vi "Format XML Parameters in Tree.vi"(7 "Path  Array IN":string[](array[string]), 8 "error in (no error)":errorcluster, 9 "Current path index":i32, 10 "Newly Added Tag":string, 11 "Tree Refnum":refnum<vi>) -> ()   [LabVIEW 2012]
doc: "SciScan 1.2 160622"
panel:
  out "error out":errorcluster
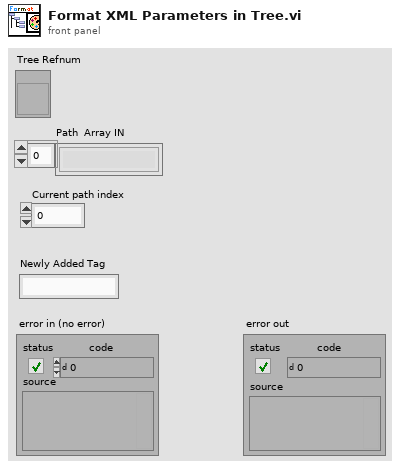
[diagram p1: front panel]
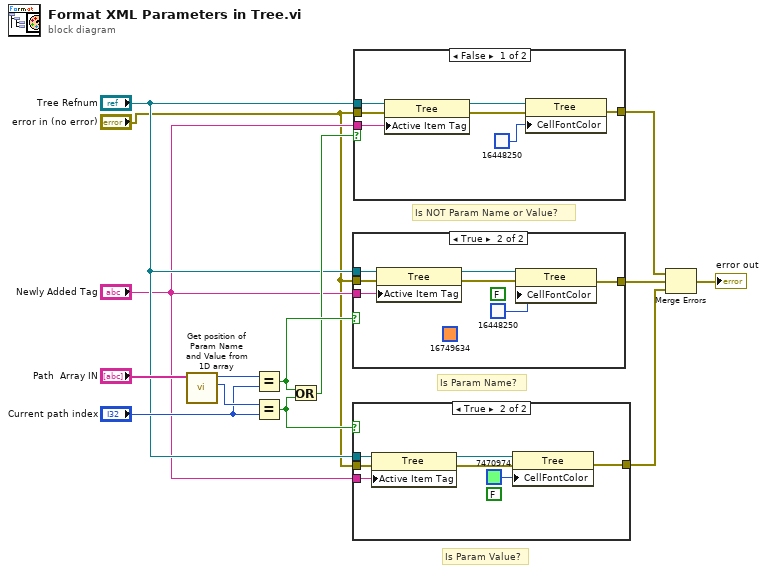
[diagram p0: block diagram]
diagram:
  # "Is NOT Param Name or Value?"
  # "Is Param Name?"
  # "Is Param Value?"
  n1 = call "Get position of Param Name and Value from 1D array.vi"("1D path array"="Path  Array IN") -> ("Index of Param Value"=w12:i32, "Index of Param Name"=w13:i32)  [unwired: 9 in]
  n2 = Equal?(x=w13, y="Current path index") -> (x = y?=w10:bool)
  n3 = Equal?(x=w12, y="Current path index") -> (x = y?=w9:bool)
  n4 = Or(x=w10, y=w9) -> (x .or. y?=w8:bool)
  n5 = case shown="True" w10 {
    tunnel: "Tree Refnum" -> [_ w22]
    tunnel: "Newly Added Tag" -> [_ w21]
    tunnel: "error in (no error)" -> [w15 w20]
    tunnel: [w15 w19] -> w3
    frame False {
    }
    frame True {
      (unwired) u32 16749634
      (unwired) FALSE ("Active Cell:Cell Font:Italic")
      n6 = property class="Tree"(reference=w22, error in=w20, "Active Item Tag"=w21) -> (reference out=w18:refnum<vi>, error out=w17:errorcluster)
      n7 = property class="Tree"(reference=w18, error in=w17, "CellFontColor"=u32 16448250) -> (error out=w19:errorcluster)  [unwired: 1 out]
    }
  }
  n8 = case shown="True" w9 {
    tunnel: "Newly Added Tag" -> [_ w30]
    tunnel: "Tree Refnum" -> [_ w29]
    tunnel: "error in (no error)" -> [w23 w25]
    tunnel: [w23 w24] -> w2
    frame False {
    }
    frame True {
      (unwired) FALSE ("Active Cell:Cell Font:Italic")
      n9 = property class="Tree"(reference=w29, error in=w25, "Active Item Tag"=w30) -> (reference out=w28:refnum<vi>, error out=w27:errorcluster)
      n10 = property class="Tree"(reference=w28, error in=w27, "CellFontColor"=u32 7470974) -> (error out=w24:errorcluster)  [unwired: 1 out]
    }
  }
  n11 = case shown="False" w8 {
    tunnel: "Newly Added Tag" -> [w37 _]
    tunnel: "Tree Refnum" -> [w36 _]
    tunnel: "error in (no error)" -> [w32 w38]
    tunnel: [w31 w38] -> w4
    frame False {
      n12 = property class="Tree"(reference=w36, error in=w32, "Active Item Tag"=w37) -> (reference out=w35:refnum<vi>, error out=w34:errorcluster)
      n13 = property class="Tree"(reference=w35, error in=w34, "CellFontColor"=u32 16448250) -> (error out=w31:errorcluster)  [unwired: 1 out]
    }
    frame True {
    }
  }
  n14 = Merge Errors(w4, w3, w2) -> (→"error out":errorcluster)
